vi "Comparison_Decision.vi"(9 "decision":dbl[](array[numeric]), 10 "SWLDA":dbl[](array[numeric]), 11 "EPR_발생_total":i16[](array[numeric])) -> (3 "selected":i32)   [LabVIEW 2014]
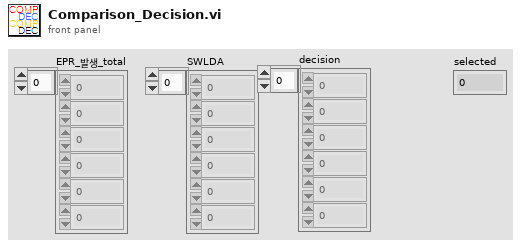
[diagram p1: front panel]
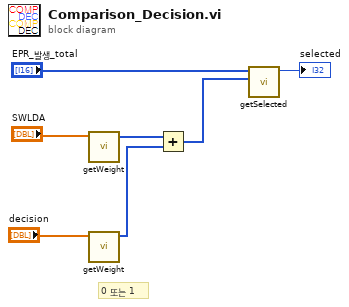
[diagram p0: block diagram]
diagram:
  # "0 또는 1"
  n1 = call "getWeight.vi"("Array"="SWLDA") -> ("Weight"=w7:i32[])  [unwired: 10 in]
  n2 = call "getWeight.vi"("Array"="decision") -> ("Weight"=w6:i32[])  [unwired: 10 in]
  n3 = Add(x=w7, y=w6) -> (x+y=w4:i32[])
  n4 = call "getSelected.vi"("Weight"=w4, "Predict"="EPR_발생_total") -> ("selected"=→"selected":i32)  [unwired: 9 in]
